vi "initialize_thread.vi"(6 "done?":bool, 8 "error in":errorcluster, 9 "this state":refnum<data-value>, 10 "parent state":refnum<data-value>, 11 "root state":refnum<data-value>) -> (0 "error out":errorcluster, 3 "Lua for LabVIEW.lvlib:Lua Thread.lvclass":refnum<class "Lua Thread.lvclass">)   [LabVIEW 2020, in "Lua for LabVIEW.lvlib" / "Lua.lvclass"]
uses:
  Lua.lvclass
  Lua Thread/Lua Thread.lvclass
  C:/Users/Nicholas Folse/Documents/workspace/github-tauterra.llc/Lua for LabVIEW/Lua for LabVIEW/Lua/Lua.lvclass
  private/lua_monitor_event.ctl
  Lua.lvclass/Lua.ctl
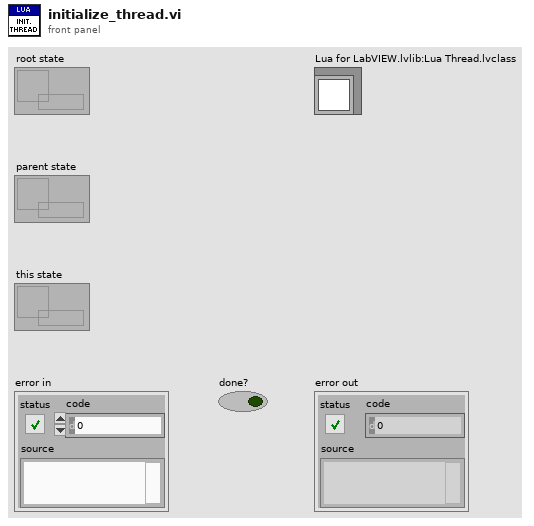
[diagram p1: front panel]
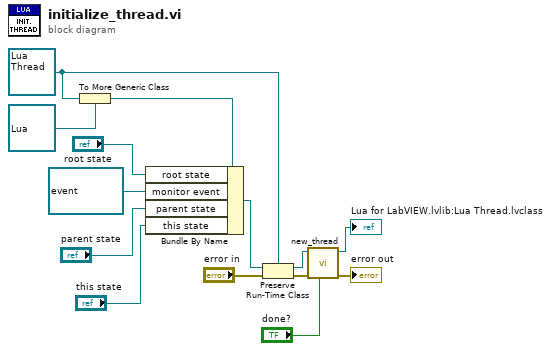
[diagram p0: block diagram]
diagram:
  w10 = refnum<class "Lua Thread.lvclass"> refnum ("Lua for LabVIEW.lvlib:Lua Thread.lvclass")
  w14 = refnum<user-event> refnum items=["<null>", "terminate"] ("monitor event")
  n1 = To More Generic Class(target class=refnum<class "Lua.lvclass"> refnum ("Lua for LabVIEW.lvlib:Lua"), reference=w10) -> (generic class reference=w12:refnum<class "Lua.lvclass">)
  n2 = Bundle By Name(cluster=w12, "root state"="root state", "monitor event"=w14, "parent state"="parent state", "this state"="this state") -> (w9:refnum<class "Lua.lvclass">)
  n3 = Preserve Run-Time Class(object in=w9, error in="error in", 2:w10) -> (object out=w5:refnum<class "Lua Thread.lvclass">, error out=w3:errorcluster)
  n4 = call "new_thread.vi"("done?"="done?", "error in (no error)"=w3, "Lua Thread in"=w5) -> ("error out"=→"error out":errorcluster, "Lua Thread out"=→"Lua for LabVIEW.lvlib:Lua Thread.lvclass":refnum<class "Lua Thread.lvclass">)  [unwired: 7 in]
